vi "Extract Excel.vi"() -> ()   [LabVIEW 2011]
uses:
  <vilib>/Utility/file.llb/Read From Spreadsheet File (string).vi
panel:
  out "Array 2":string[](array[string])
  out "Array":string[](array[string])
  out "all rows":string[][](array[string])
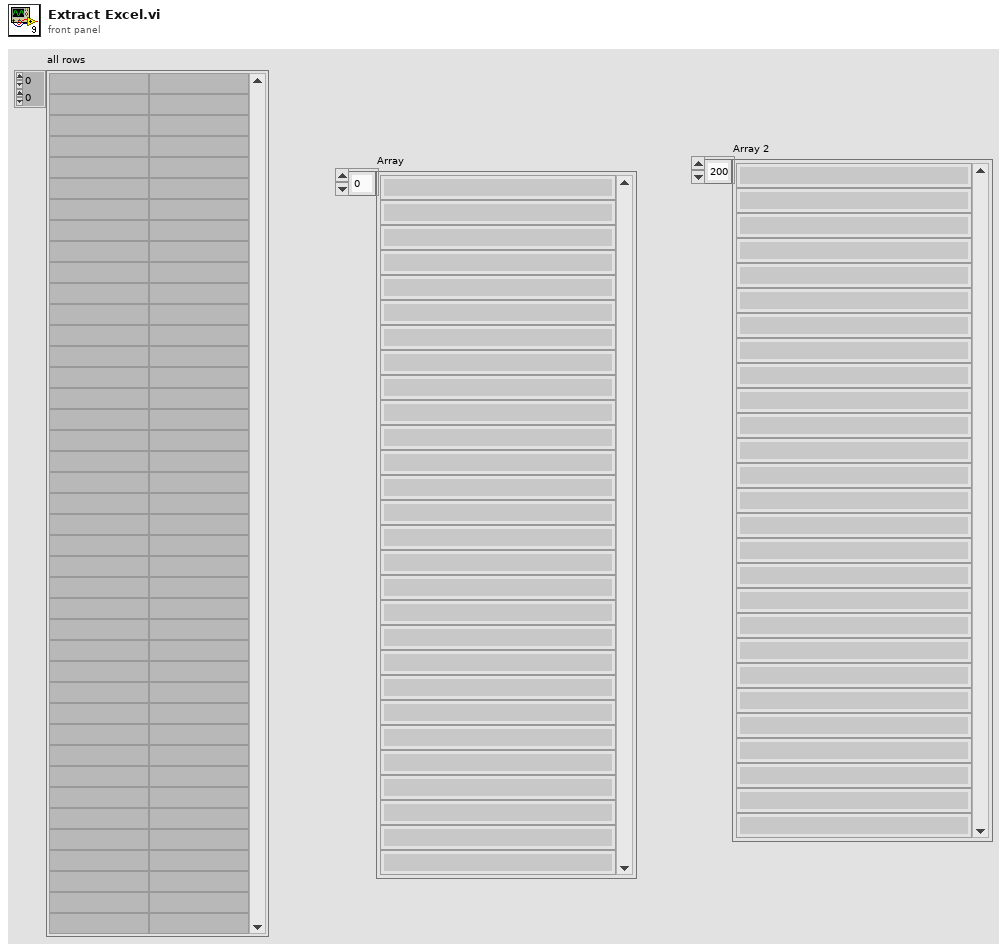
[diagram p1: front panel]
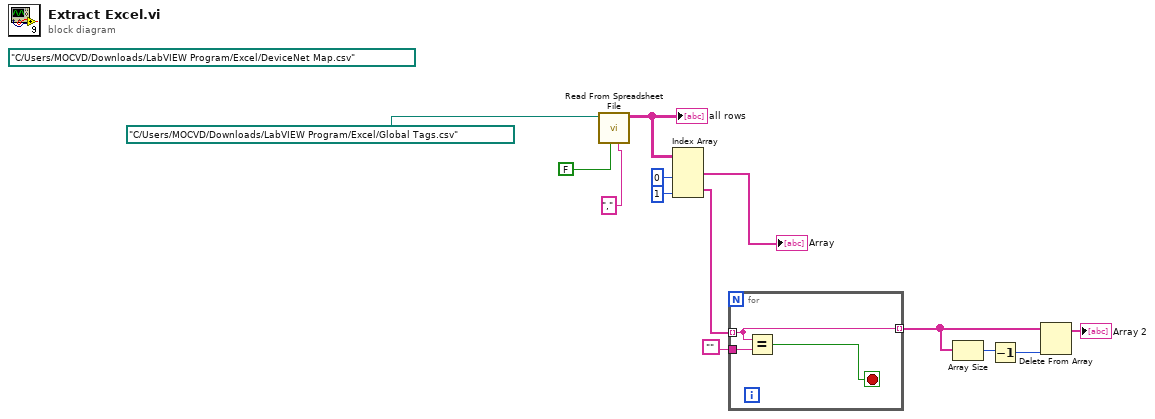
[diagram p0: block diagram]
diagram:
  (unwired) path "C:/Users/MOCVD/Downloads/LabVIEW Program/Excel/DeviceNet Map.csv"
  n1 = call-poly <vilib>:"Read From Spreadsheet File.vi"("delimiter (\\t)"=",", "transpose (no:F)"=FALSE, "file path (dialog if empty)"=path "C:/Users/MOCVD/Downloads/LabVIEW Program/Excel/Global Tags.csv") -> ("all rows"=w10:string[][])  [unwired: 4 in, 4 out]
  "all rows" <- w10
  n2 = Index Array(array=w10, index (col) #1=0 ("disabled index (col)"), index (col) #2=1 ("index (col)")) -> (element #1=→"Array":string[], element #2=w6:string[])  [unwired: 2 in]
  n3 = for {
    tunnel: w6 -> [w14] mode=indexing
    tunnel: "" -> [w16]
    tunnel: [w14] -> w4 mode=indexing
    stop <- w15 stop-if-true
    n4 = Equal?(x=w14, y=w16) -> (x = y?=w15:bool)
  }
  n5 = Array Size(array=w4) -> (size(s)=w3:i32)
  n6 = Decrement(x=w3) -> (x-1=w2:i32)
  n7 = Delete From Array(array=w4, index=w2) -> (array with subset deleted=→"Array 2":string[])  [unwired: 1 in, 1 out]
